vi "i2clib_close.vi"(8 "error in (no error)":errorcluster, 11 "I2C Reference":i32) -> (0 "error out":errorcluster)   [LabVIEW 2017]
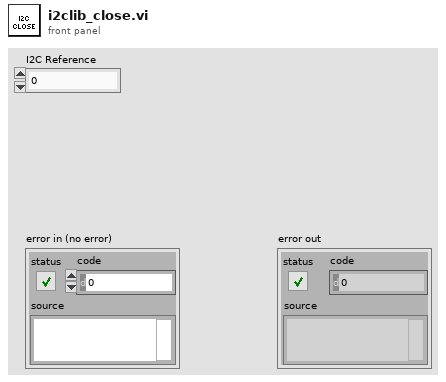
[diagram p1: front panel]
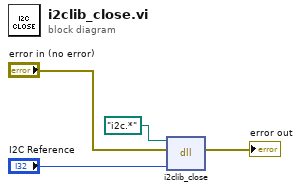
[diagram p0: block diagram]
diagram:
  n1 = dll-call lib="?" fn="i2clib_close"(path in=path "i2c.*", error in="error in (no error)", "handle"="I2C Reference") -> (error out=→"error out":errorcluster)  [unwired: 3 in, 1 out]
